vi "Manual Mode.vi"(8 "error in (no error)":errorcluster, 10 "Test Settings":T1, 11 "Context in":refnum<class "Context.lvclass">) -> (0 "error out":errorcluster, 3 "Context out":refnum<class "Context.lvclass">)   [LabVIEW 2016, in "Context.lvclass"]
uses:
  Context.lvclass
  Typedefs/TestSettings.ctl
  Context.lvclass/Context.ctl
  States/State/State.lvclass
  Model/Model/Model.lvclass
  Typedefs/HPMT_Typedefs.lvlib
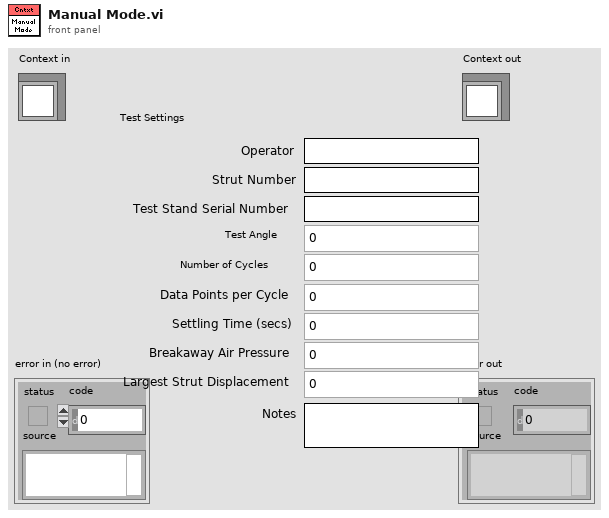
[diagram p1: front panel]
types:
  T1 = typedef "HPMT_Typedefs.lvlib/TestSettings.ctl" = cluster{"Operator":string, "Strut Number":string, "Test Stand Serial Number":string, "Notes":string, "Test Angle":u16, "Number of Cycles":u16, "Data Points per Cycle":u16, "Settling Time (secs)":u16, "Breakaway Air Pressure":u16, "Largest Strut Displacement":dbl}
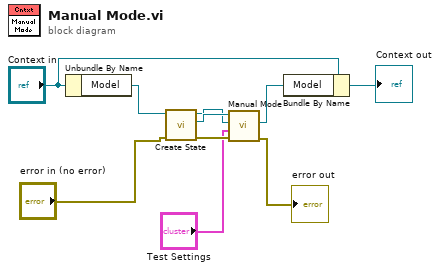
[diagram p0: block diagram]
diagram:
  n1 = Unbundle By Name("Context in") -> ("Model"=w10:refnum<class "Model.lvclass">)
  n2 = call "Create State.vi"("error in (no error)"="error in (no error)", "Model in"=w10) -> ("error out"=w6:errorcluster, "State"=w8:refnum<class "State.lvclass">, "Model out"=w7:refnum<class "Model.lvclass">)  [unwired: 7 in]
  n3 = call-dynamic "Manual Mode.vi"("error in (no error)"=w6, "Test Settings"="Test Settings", "Model in"=w7, "State in"=w8) -> ("error out"=→"error out":errorcluster, "Model out"=w3:refnum<class "Model.lvclass">)  [unwired: 5 in, 1 out]
  n4 = Bundle By Name(cluster="Context in", "Model"=w3) -> (→"Context out":refnum<class "Context.lvclass">)
